vi "EventLog.ExtendError.vi"(7 "Source (All)":T1, 8 "error in":errorcluster, 10 "ErrData":T2) -> (0 "error out":errorcluster)   [LabVIEW 2013]
uses:
  EventLog.EventLevel.ctl
  Translator/Translator.Message.ctl
  EventLog.EventGui.ctl
  EventLog.Buffer.Action.ctl
  EventLog.Event.ctl
  Global/ApplicationGlobal.vi
  User/User.Global.vi
  EventLog.EventSource.ctl
  CitTemplate/citTemplate.errData.ctl
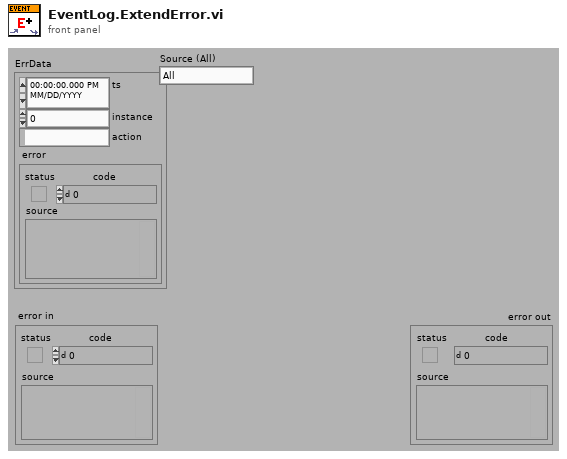
[diagram p1: front panel]
types:
  T1 = typedef "EventLog.EventSource.ctl" = enum16{"All", "Gui", "Ref", "DB", "Seq", "File", "DIO", "AI", "AO", "Barcode", "CPX"}
  T2 = typedef "citTemplate.errData.ctl" = cluster{"ts":timestamp, "instance":i32, "action":string, "error":errorcluster}
  T3 = typedef "Translator.Message.ctl" = enum16{"-", "Event confirmed", "Log out", "Log in", "Shutdown", "Cancel", "Start", "Error %d >> %s", "Error %d >> %s >> %s", "Starting %s", "Quitting %s", "User %s level %s added", "User %s level %s deleted", "User %s level %s changed to %s", "Configured", "Initializing", "Quitting", "Loading", "Running", "Stopped", "Do you want to continue?", "Calibration", "Log out?", "System", "All", "IDLE", "Translating...%s", "Not found", "Alarm %s", "Restart is required to translate the application! Do you want to restart the PC?", "Restart cancelled. Be aware that some controls may not be fully translated until you restart the application.", "New version available!", "The software is up-to-date", "PC software will be updated after rebooting the PC. Do you want to reboot now?", "RT software will be updated. Make sure that no process is running. Do you want to reboot RT now?", "Updating RT firmware. Please wait...", "Update failed: %s", "Rebooting...", "Rebooting RT. Please wait...", "RT updated to version %s", "Timeout error during update. Check if RT is working", "Run", "Skip", "Abort", "Please wait...", "Database disconnected - changeover disabled!", "Put reference number...", "Folder '%s' is missing", "File '%s' is missing", "File '%s' is broken", "File '%s' is running", "Log file '%s' started", "Step '%s' added to log file", "Log file '%s' ended", "Test steps are missing", "Output %s = %.3f", "Process param '%s' not found in DB", "Process param '%s' wrong order", "Process param '%s' value %.3f out of limits (%.3f; %.3f)", "Step%d param '%s' not found in DB", "Step%d param '%s' wrong order", "Step%d param '%s' value %.3f out of limits (%.3f; %.3f)", "Step%d EV '%s' not found in DB", "Step%d EV '%s' wrong order", "Get steps for reference '%s'", "Scan label failed", "Scan label failed. Error %d", "Scan label failed. Scanner disconnected", "Scan label: %s, %s", "Scan plate failed", "Scan plate failed. Wrong reference %s", "Scan plate failed. Error %s", "Scan plate failed. Scanner disconnected", "Scan plate: %s"}
  T4 = typedef "EventLog.Event.ctl" = cluster{"ts":dbl, "lev":T5, "usr":i32, "src":T1, "msg":T3, "arg":variant[]}
  T5 = typedef "EventLog.EventLevel.ctl" = enum8{"Debug", "Info", "Warning", "Error"}
  T6 = typedef "EventLog.Buffer.Action.ctl" = enum16{"init", "re-init", "clear", "set translator", "add", "get"}
  T7 = typedef "EventLog.EventGui.ctl" = cluster{"ts":dbl, "lev":T5, "usr":i32, "src":T1, "msg":T3, "arg":variant[], "msg_str":string}
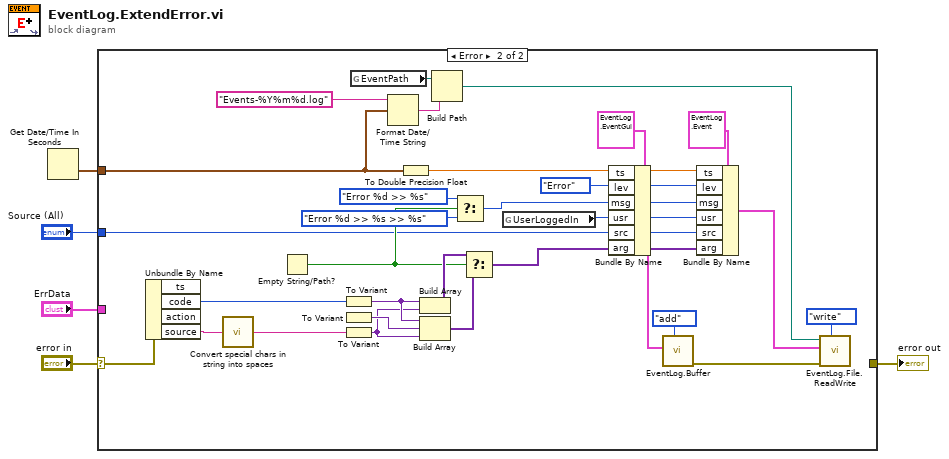
[diagram p0: block diagram]
diagram:
  n1 = Get Date/Time In Seconds() -> (seconds since 1Jan1904=w1:timestamp)
  n2 = case shown="Error" "error in" {
    selector: "error in" -> [w6 w8]
    tunnel: [w6 _] -> w5
    tunnel: "ErrData" -> [_ _]
    tunnel: "Source (All)" -> [_ w12]
    tunnel: w1 -> [_ w7]
    frame No Error {
    }
    frame Error {
      w10 = EventLog.EventLevel."Error" ("lev")
      n3 = Unbundle By Name(w8) -> ("code"=w23:i32, "source"=w25:string)  [unwired: 2 out]
      n4 = call "Convert special chars in string into spaces.vi"("string with special characters"=w25) -> ("string with spaces"=w24:string)  [unwired: 2 in]
      n5 = Empty String/Path?() -> (empty?=w14:bool)  [unwired: 1 in]
      n6 = To Variant(anything=w23) -> (Variant=w21:variant)
      n7 = To Variant() -> (Variant=w20:variant)  [unwired: 1 in]
      n8 = To Variant(anything=w24) -> (Variant=w19:variant)
      n9 = global read "ApplicationGlobal.vi" "EventPath"() -> (w29:path)
      n10 = Format Date/Time String(time format string (%c)="Events-%Y%m%d.log", seconds (now)=w7) -> (date/time string=w28:string)  [unwired: 1 in]
      n11 = To Double Precision Float(number=w7) -> (double precision float=w32:dbl)
      n12 = Build Array(w21, w19) -> (w22:variant[])
      n13 = Build Array(w21, w20, w19) -> (w18:variant[])
      n14 = Build Path(base path=w29, name or relative path=w28) -> (appended path=w27:path)
      n15 = Select(t=Translator.Message."Error %d >> %s" ("msg"), s=w14, f=Translator.Message."Error %d >> %s >> %s" ("msg")) -> (s? t:f=w13:T3)
      n16 = Select(t=w22, s=w14, f=w18) -> (s? t:f=w17:variant[])
      n17 = global read "User.Global.vi" "UserLoggedIn"() -> (w26:i32)
      n18 = Bundle By Name(cluster=T7 {"ts"=0.0, "lev"=enum."Debug", "usr"=0, "src"=enum."All", "msg"=enum."Log out", "arg"=[], "msg_str"=""} ("Event in"), "ts"=w32, "lev"=w10, "msg"=w13, "usr"=w26, "src"=w12, "arg"=w17) -> (w11:T7)
      n19 = call "EventLog.Buffer.vi"("action (get)"=EventLog.Buffer.Action."add" ("action (read)"), "Event in"=w11) -> ("error out"=w9:errorcluster)  [unwired: 6 in, 3 out]
      n20 = Bundle By Name(cluster=T4 {"ts"=0.0, "lev"=enum."Debug", "usr"=0, "src"=enum."All", "msg"=enum."Log out", "arg"=[]} ("event in"), "ts"=w32, "lev"=w10, "msg"=w13, "usr"=w26, "src"=w12, "arg"=w17) -> (w31:T4)
      n21 = call "EventLog.File.ReadWrite.vi"("action (read)"=enum16{"read", "write"}."write", "error in"=w9, "event in"=w31, "file"=w27) -> ()  [unwired: 3 in, 5 out]
    }
  }
  "error out" <- w5
